vi "CreateSensorSession.vi"(8 "error in (no error)":errorcluster, 11 "RoomAlert in":refnum<class "RoomAlert.lvclass">) -> (0 "error out":errorcluster, 3 "RoomAlert out":refnum<class "RoomAlert.lvclass">)   [LabVIEW 2018, in "SensorPlugins.lvlib" / "RoomAlert.lvclass"]
doc: "Opens a communication link between the application and the RoomAlert Device using the Port number."
uses:
  RoomAlert.lvclass
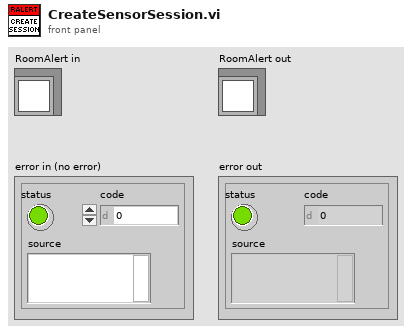
[diagram p1: front panel]
types:
  T1 = typedef "SensorPlugins.lvlib/RoomAlert.lvclass/RoomAlertControls.ctl" = cluster{"Connected?":bool, "IP Address of SNMP Device":string, "Port (161)":u16, "Community Name":string, "Measurements To Read Array":u16[], "Update Light \nTower?":bool, "LightTower":cluster{"Red":bool, "Amber":bool, "Green":bool, "Audio":bool}}[]
  T2 = typedef "SensorPlugins.lvlib/RoomAlert.lvclass/CommunicationControls.ctl" = refnum<k16>[]
  T3 = cluster{"Connected?":bool, "IP Address of SNMP Device":string, "Port (161)":u16, "Community Name":string, "Measurements To Read Array":u16[], "Update Light \nTower?":bool, "LightTower":cluster{"Red":bool, "Amber":bool, "Green":bool, "Audio":bool}}
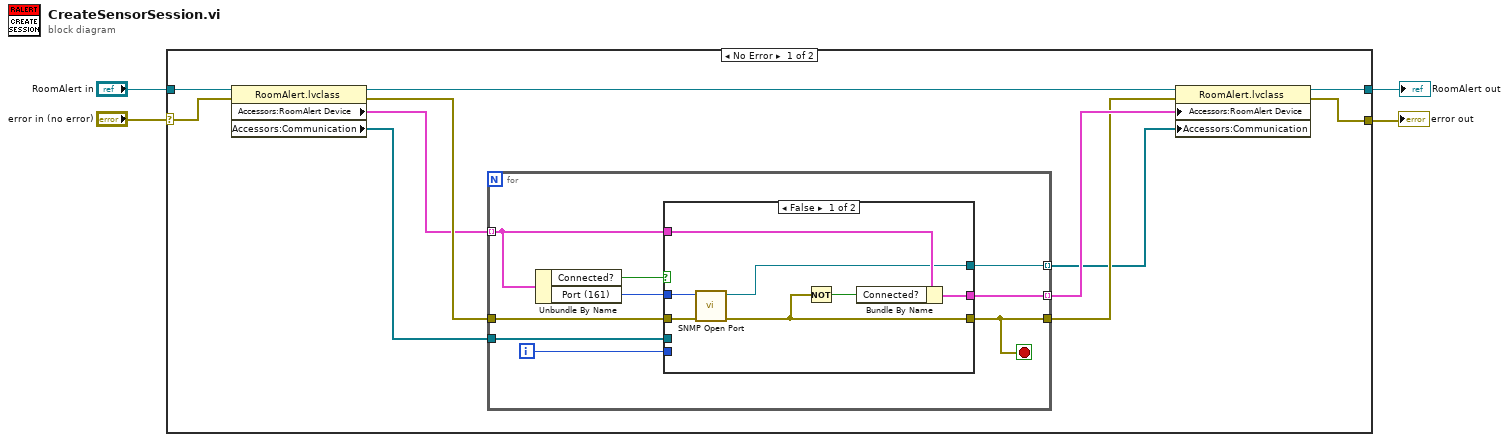
[diagram p0: block diagram]
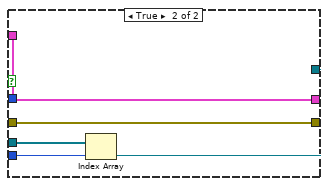
[diagram p2: hidden frame]
diagram:
  n1 = case shown="No Error" "error in (no error)" {
    selector: "error in (no error)" -> [w14 w37]
    tunnel: "RoomAlert in" -> [w15 w38]
    tunnel: [w11 w38] -> w2
    tunnel: [w7 w37] -> w1
    frame No Error {
      n2 = property class="RoomAlert.lvclass"(reference=w15, error in=w14) -> (reference out=w10:refnum<class "RoomAlert.lvclass">, error out=w13:errorcluster, "Accessors:RoomAlert Device"=w12:T1, "Accessors:Communication "=w5:T2)
      n3 = for {
        tunnel: w13 -> [w22]
        tunnel: [w21] -> w8
        tunnel: w12 -> [w24] mode=indexing
        tunnel: [w23] -> w9 mode=indexing
        tunnel: [w16] -> w6 mode=indexing
        tunnel: w5 -> [w17]
        i -> [w18]
        stop <- w21 stop-if-true
        n4 = Unbundle By Name(w24) -> ("Connected?"=w19:bool, "Port (161)"=w20:u16)
        n5 = case shown="False" w19 {
          tunnel: w24 -> [w31 w36]
          tunnel: [w30 w36] -> w23
          tunnel: w22 -> [w28 w35]
          tunnel: [w27 w35] -> w21
          tunnel: [w25 w32] -> w16
          tunnel: w20 -> [w26 _]
          tunnel: w18 -> [_ w34]
          tunnel: w17 -> [_ w33]
          frame False {
            n6 = call "SNMP Open Port.vi"("error in (no error)"=w28, "port"=w26) -> ("error out"=w27:errorcluster, "connection ID"=w25:refnum<k16>)  [unwired: 8 out]
            n7 = Not(x=w27) -> (.not. x?=w29:bool)
            n8 = Bundle By Name(cluster=w31, "Connected?"=w29) -> (w30:T3)
          }
          frame True {
            n9 = Index Array(array=w33, index=w34) -> (element=w32:refnum<k16>)
          }
        }
      }
      n10 = property class="RoomAlert.lvclass"(reference=w10, error in=w8, "Accessors:RoomAlert Device"=w9, "Accessors:Communication "=w6) -> (reference out=w11:refnum<class "RoomAlert.lvclass">, error out=w7:errorcluster)
    }
    frame Error {
    }
  }
  "error out" <- w1
  "RoomAlert out" <- w2
